vi "proje.vi"() -> ()   [LabVIEW 2017]
uses:
  <vilib>/MakerHub/LINX/Public/Peripherals/Analog/Analog Read 1 Chan.vi
  <vilib>/MakerHub/LINX/Public/Peripherals/Analog/Analog Read N Chans.vi
  <vilib>/MakerHub/LINX/Private/Local IO/LinxAnalogRead.vi
  <vilib>/MakerHub/LINX/Public/Utilities/Check Channel.vi
  <vilib>/MakerHub/LINX/Public/Utilities/Open Serial.vi
  <vilib>/MakerHub/LINX/Private/Utilties/Generate Error.vi
  <vilib>/MakerHub/LINX/LMH-LINX.lvlib
panel:
  out "Voltage":dbl
  in  "Baud Rate Override":u32
  in  "Dur":bool
  in  "Serial Port":refnum<visa-resource-name>="N/A"
  out "Iþýk Seviyesi":u8(slide) scale=0.0..100.0
  out "Thermometer":dbl(slide) scale=0.0..100.0
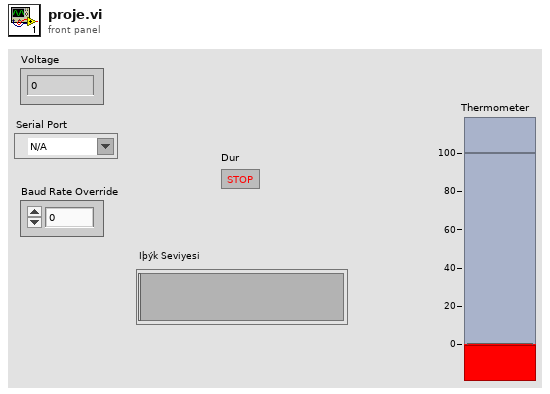
[diagram p1: front panel]
types:
  T1 = typedef "LMH-LINX.lvlib/LINX Ref.ctl" = cluster{"IO":T2, "Interface":T3, "LINX Device Config":T4}
  T2 = typedef "LMH-LINX.lvlib/Platform.ctl" = enum16{"Remote", "Local"}
  T3 = typedef "LMH-LINX.lvlib/Interface.ctl" = enum16{"Serial", "TCP"}
  T4 = typedef "LMH-LINX.lvlib/Device.lvlib/LINX Device Config.ctl" = cluster{"Interface":T3, "COM Port":refnum<visa-resource-name>, "TCP Configuration":T5, "Device Family":u8, "Device ID":u8, "Device Name":string, "TCP Ref":refnum<k5>, "Channels":T6}
  T5 = typedef "LMH-LINX.lvlib/Device.lvlib/TCP Config.ctl" = cluster{"IP Address":string, "Port":u16}
  T6 = typedef "LMH-LINX.lvlib/Channels.ctl" = cluster{"DI":u8[], "DO":u8[], "AI":u8[], "AO":u8[], "PWM":u8[], "QE":u8[], "UART":u8[], "I2C 2":u8[], "SPI":u8[], "CAN":u8[], "Servo":u8[], "AI Ref (V)":dbl, "AI Resolution (Bits)":u8, "AO Ref (V)":dbl, "AO Resolution (Bits)":u8}
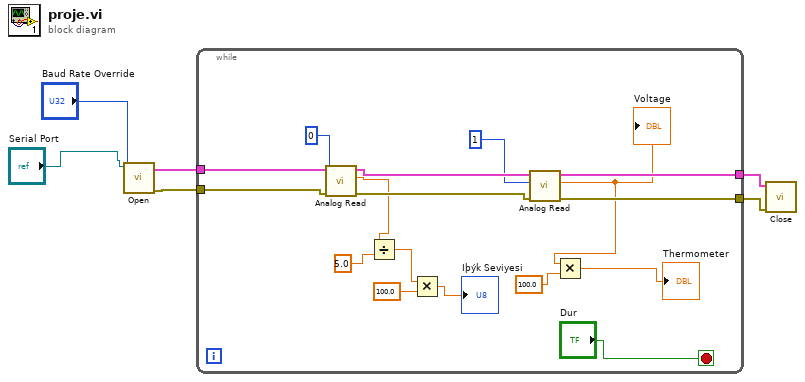
[diagram p0: block diagram]
diagram:
  n1 = call-poly <vilib>:"Open.vi"("Baud Rate Override"="Baud Rate Override", "Serial Port"="Serial Port") -> ("Error Out"=w6:errorcluster, "LINX Resource"=w5:T1)  [unwired: 7 in, 1 out]
  n2 = while {
    tunnel: w6 -> [w18]
    tunnel: w5 -> [w17]
    tunnel: [w13] -> w4
    tunnel: [w12] -> w3
    stop <- "Dur" stop-if-true
    n3 = call-poly <vilib>:"Analog Read.vi"("Error In"=w18, "Analog Channel"=u8 0, "LINX Resource"=w17) -> ("Error Out"=w15:errorcluster, "Voltage"=w14:dbl, "LINX Resource"=w16:T1)  [unwired: 5 in, 1 out]
    n4 = Divide(x=w14, y=5.0) -> (x/y=w22:dbl)
    n5 = Multiply(x=w22, y=100.0) -> (x*y=→"Iþýk Seviyesi":dbl)
    n6 = call-poly <vilib>:"Analog Read.vi"("Error In"=w15, "Analog Channel"=u8 1, "LINX Resource"=w16) -> ("Error Out"=w12:errorcluster, "Voltage"=w8:dbl, "LINX Resource"=w13:T1)  [unwired: 5 in, 1 out]
    "Voltage" <- w8
    n7 = Multiply(x=w8, y=100.0) -> (x*y=→"Thermometer":dbl)
  }
  n8 = call <vilib>:"Close.vi"("Error In"=w3, "LINX Resource"=w4) -> ()  [unwired: 9 in, 1 out]
